vi "Get Post.vi"(8 "error in (no error)":errorcluster, 10 "id":i32, 11 "My API in":refnum<class "My API.lvclass">) -> (0 "error out":errorcluster, 2 "Post":T1, 3 "My API out":refnum<class "My API.lvclass">)   [LabVIEW 2017, in "My API.lvclass"]
uses:
  My API.lvclass
  Post.ctl
  My API.lvclass/My API.ctl
  classes/REST Client/REST Client.lvclass
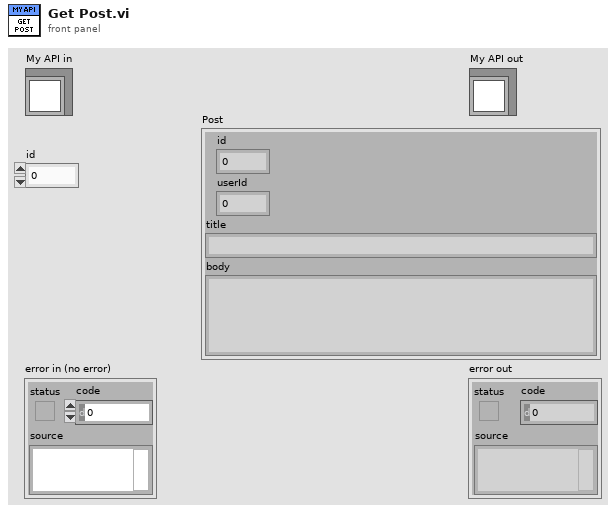
[diagram p1: front panel]
types:
  T1 = typedef "My API.lvclass/Post.ctl" = cluster{"id":i32, "userId":i32, "title":string, "body":string}
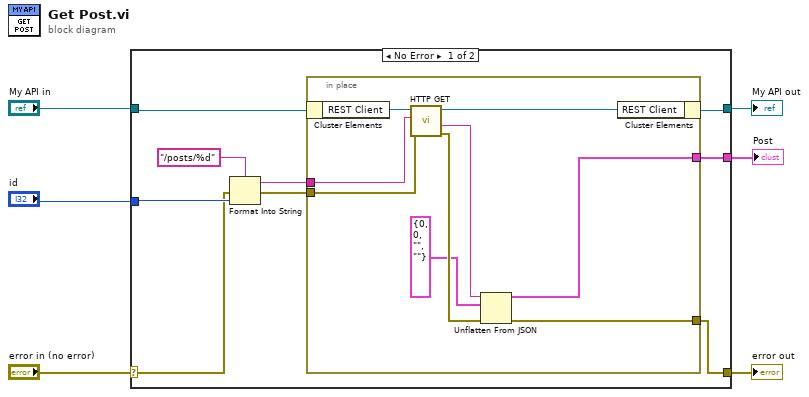
[diagram p0: block diagram]
diagram:
  n1 = case shown="No Error" "error in (no error)" {
    selector: "error in (no error)" -> [w13 w26]
    tunnel: [w9 w26] -> w5
    tunnel: [w7 w25] -> w3
    tunnel: "My API in" -> [w12 w25]
    tunnel: "id" -> [w14 _]
    tunnel: [w8 _] -> w1
    frame No Error {
      n2 = Format Into String(format string="/posts/%d", error in=w13, w14) -> (resulting string=w11:string, error out=w10:errorcluster)  [unwired: 1 in]
      n3 = in-place {
        in-place-border: w11 -> [w23]
        in-place-border: w10 -> [w22]
        in-place-border: [w16] -> w9
        in-place-border: [w17] -> w8
        n4 = in-place-cluster #1(w12) -> ("REST Client"=w24:refnum<class "REST Client.lvclass">)
        n5 = call-dynamic "HTTP GET.vi"("error in (no error)"=w22, "Path"=w23, "REST Client in"=w24) -> ("error out"=w19:errorcluster, "Response body"=w21:string, "REST Client out"=w20:refnum<class "REST Client.lvclass">)  [unwired: 3 in, 3 out]
        n6 = Unflatten From JSON(JSON string=w21, type and defaults=T1 {"id"=0, "userId"=0, "title"="", "body"=""} ("Post"), error in (no error)=w19) -> (value=w17:T1, error out=w16:errorcluster)  [unwired: 4 in]
        n7 = in-place-cluster #1("REST Client"=w20) -> (w7:refnum<class "My API.lvclass">)
      }
    }
    frame Error {
    }
  }
  "error out" <- w5
  "My API out" <- w3
  "Post" <- w1
